vi "Lower_Stop_ms3_20220318end.vi"(8 "error in (no error)":errorcluster, 10 "I-O in":refnum<class "I-O.lvclass">, 11 "Motion in":refnum<class "Motion.lvclass">) -> (0 "error out":errorcluster, 2 "I-O out":refnum<class "I-O.lvclass">, 3 "Motion out":refnum<class "Motion.lvclass">)   [LabVIEW 2016]
uses:
  Classes/Controller/Motion/Motion Folder/Motion.lvclass
  Classes/Controller/I-O/I-O Folder/I-O.lvclass
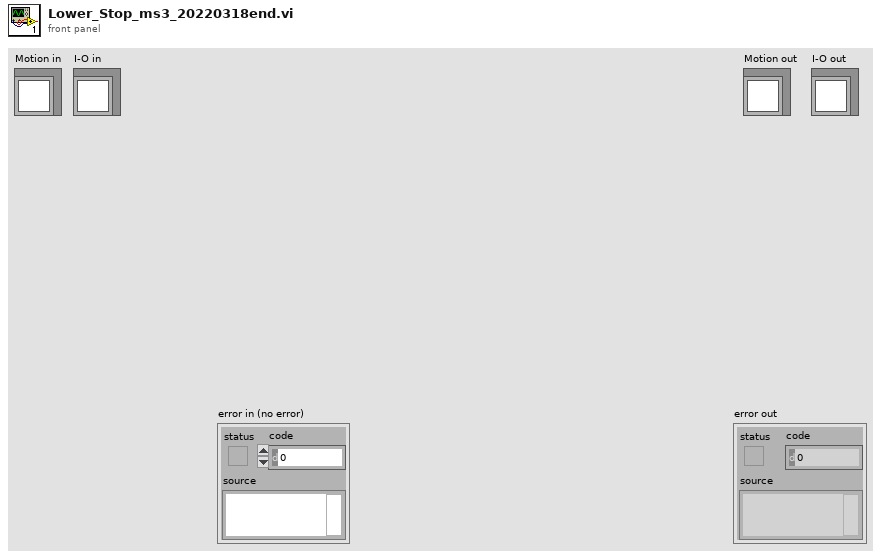
[diagram p1: front panel]
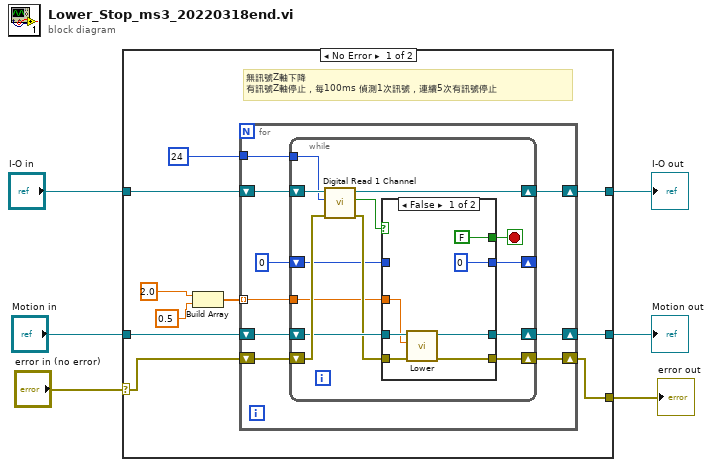
[diagram p0: block diagram]
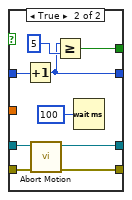
[diagram p2: hidden frame]
diagram:
  n1 = case shown="No Error" "error in (no error)" {
    selector: "error in (no error)" -> [w14 w57]
    tunnel: [w9 w57] -> w5
    tunnel: "Motion in" -> [w16 w56]
    tunnel: "I-O in" -> [w15 w55]
    tunnel: [w8 w56] -> w2
    tunnel: [w7 w55] -> w1
    frame No Error {
      # "無訊號Z軸下降\n有訊號Z軸停止，每100ms 偵測1次訊號，連續5次有訊號停止"
      n2 = Build Array(2.0 ("Speed"), 0.5 ("Speed")) -> (w10:dbl[])
      n3 = for {
        shift-right: [w17] -> w8
        shift-left: w16 -> [w25]
        shift-right: [w19] -> w7
        shift-left: w15 -> [w24]
        shift-right: [w18] -> w9
        shift-left: w14 -> [w23]
        tunnel: 24 ("Read") -> [w22]
        tunnel: w10 -> [w21] mode=indexing
        n4 = while {
          shift-right: [w33] -> w17
          shift-left: w25 -> [w36]
          shift-right: [w32] -> w19
          shift-left: w24 -> [w38]
          shift-right: [w31] -> w18
          shift-left: w23 -> [w37]
          tunnel: w22 -> [w30]
          tunnel: w21 -> [w29]
          shift-right: [w27] -> _
          shift-left: 0 -> [w28]
          stop <- w26 stop-if-true
          n5 = call-dynamic "Digital Read 1 Channel.vi"("error in (no error)"=w37, "Read"=w30, "I-O in"=w38) -> ("error out"=w34:errorcluster, "Value"=w35:bool, "I-O out"=w32:refnum<class "I-O.lvclass">)  [unwired: 6 in]
          n6 = case shown="False" w35 {
            tunnel: w36 -> [w45 w54]
            tunnel: w34 -> [w42 w53]
            tunnel: [w44 w52] -> w33
            tunnel: [w43 w51] -> w31
            tunnel: w29 -> [w41 _]
            tunnel: w28 -> [_ w49]
            tunnel: [0 w48] -> w27
            tunnel: [FALSE ("Value") w47] -> w26
            frame False {
              n7 = call-dynamic "Lower.vi"("error in (no error)"=w42, "Speed"=w41, "Motion in"=w45) -> ("error out"=w43:errorcluster, "Motion out"=w44:refnum<class "Motion.lvclass">)  [unwired: 7 in]
            }
            frame True {
              n8 = Increment(x=w49) -> (x+1=w48:i32)
              n9 = call-dynamic "Abort Motion.vi"("error in (no error)"=w53, "Motion in"=w54) -> ("error out"=w51:errorcluster, "Motion out"=w52:refnum<class "Motion.lvclass">)  [unwired: 8 in]
              n10 = Greater Or Equal?(x=w48, y=5) -> (x >= y?=w47:bool)
              n11 = Wait (ms)(milliseconds to wait=u32 100) -> ()  [unwired: 1 out]
            }
          }
        }
      }
    }
    frame Error {
    }
  }
  "error out" <- w5
  "Motion out" <- w2
  "I-O out" <- w1
